vi "DIO_task_array.vi"() -> ()   [LabVIEW 2013]
panel:
  in  "Task Array":refnum<k21>[](array[refnum])=["RemoteEnable_S3P00L0", "AirVoltageOut_S3AO0", "MethaneVoltageOut_S3AO1", "PressureVoltageIn_S3AI8", "SelectAxisOut_S3P00L1-2", "EncodePosIn_S3P1", "ReadAxisFlag_S3P00L4", "ByteReadFlag_S3P00L3", "XYmotorEnable_S3P2L1", "Xdirection_S3P2L2-3", "Ydirection_S3P2L6-7"]
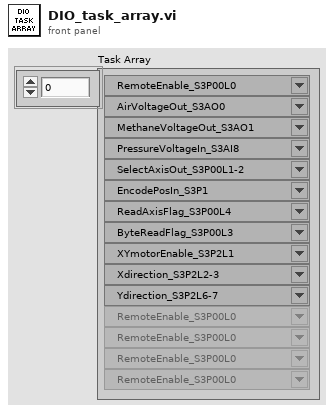
[diagram p1: front panel]
diagram:
